vi "Color_Project.vi"() -> ()   [LabVIEW 2014]
uses:
  leitura de dados txt control.ctl
panel:
  out "L*a*b*":dbl[](array[numeric])
  out "r1":dbl[](array[numeric])
  out "Reflectance2":string[][](array[string])
  out "teste":i32[](array[numeric])
  out "IL Table":string[][](array[string])
  out "ILCols":i32
  out "ILRows":i32
  out "Selected illuminant":dbl[](array[numeric])
  out "Reflectance":i32[](array[numeric])
  out "Is CMF selected?":bool
  out "Is illuminant selected?":bool
  out "Intepoled iluminants":dbl[][](array[numeric])
  out "Selected\nCMF":dbl[][](array[numeric])
  out "cmf Index":dbl
  out "CMFCols":i32
  out "CMFRows":i32
  out "CMF Table":string[][](array[string])
  in  "Color Matching Function":string(combo)
  out "Illuminant Graph":T1(graph)
  out "LambdaInterval":dbl[](array[numeric])
  out "NeedInterpolation?":bool
  out "Selected illuminant index":dbl
  in  "Select Illuminant":T2
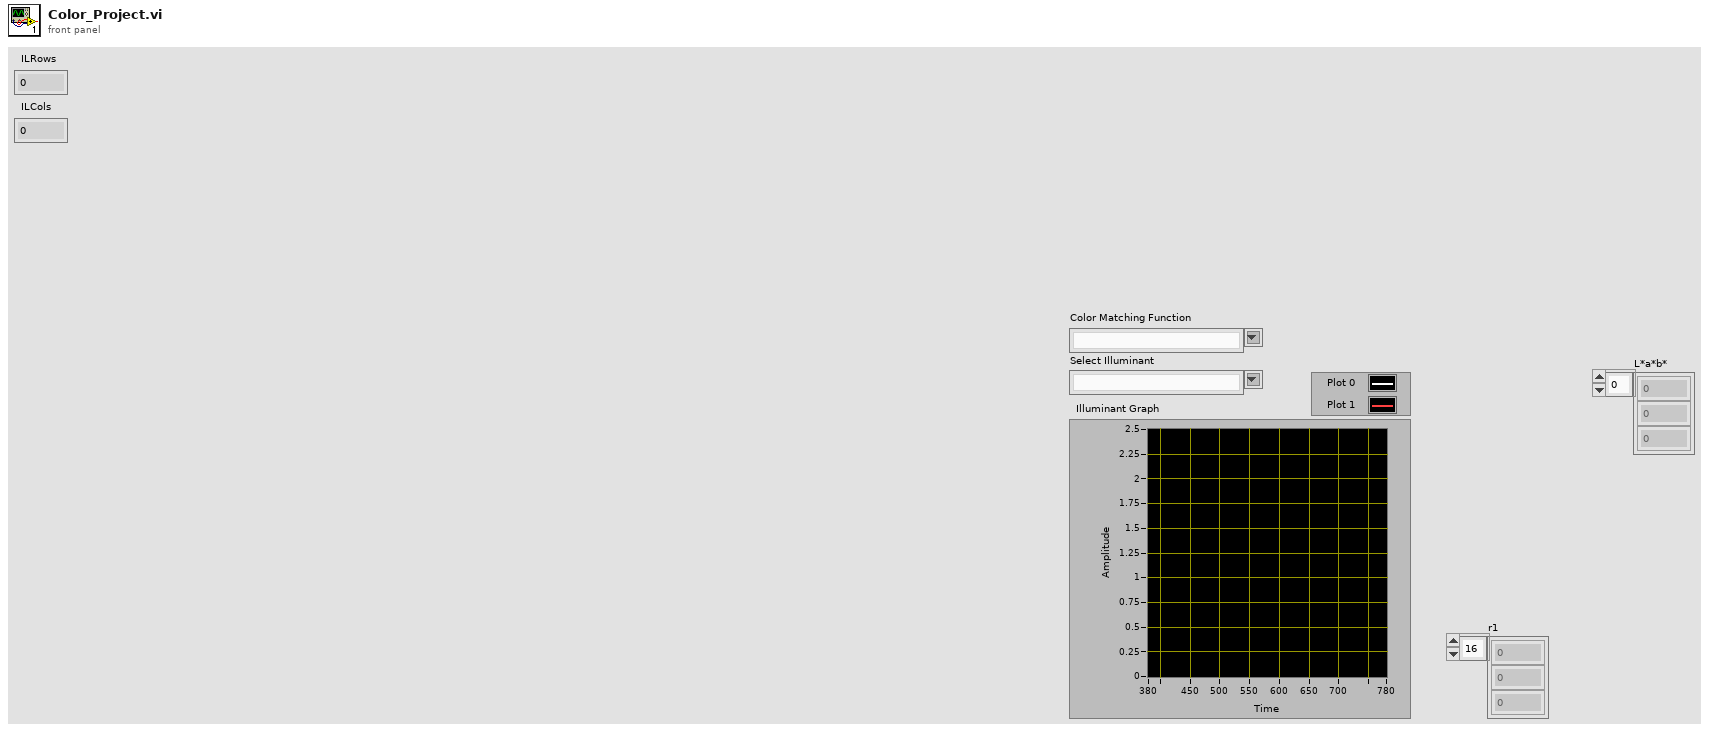
[diagram p1: front panel]
types:
  T1 = cluster{"GammaInterval":dbl[], "Interpolated":dbl[]}[]
  T2 = typedef "leitura de dados txt control.ctl" = string
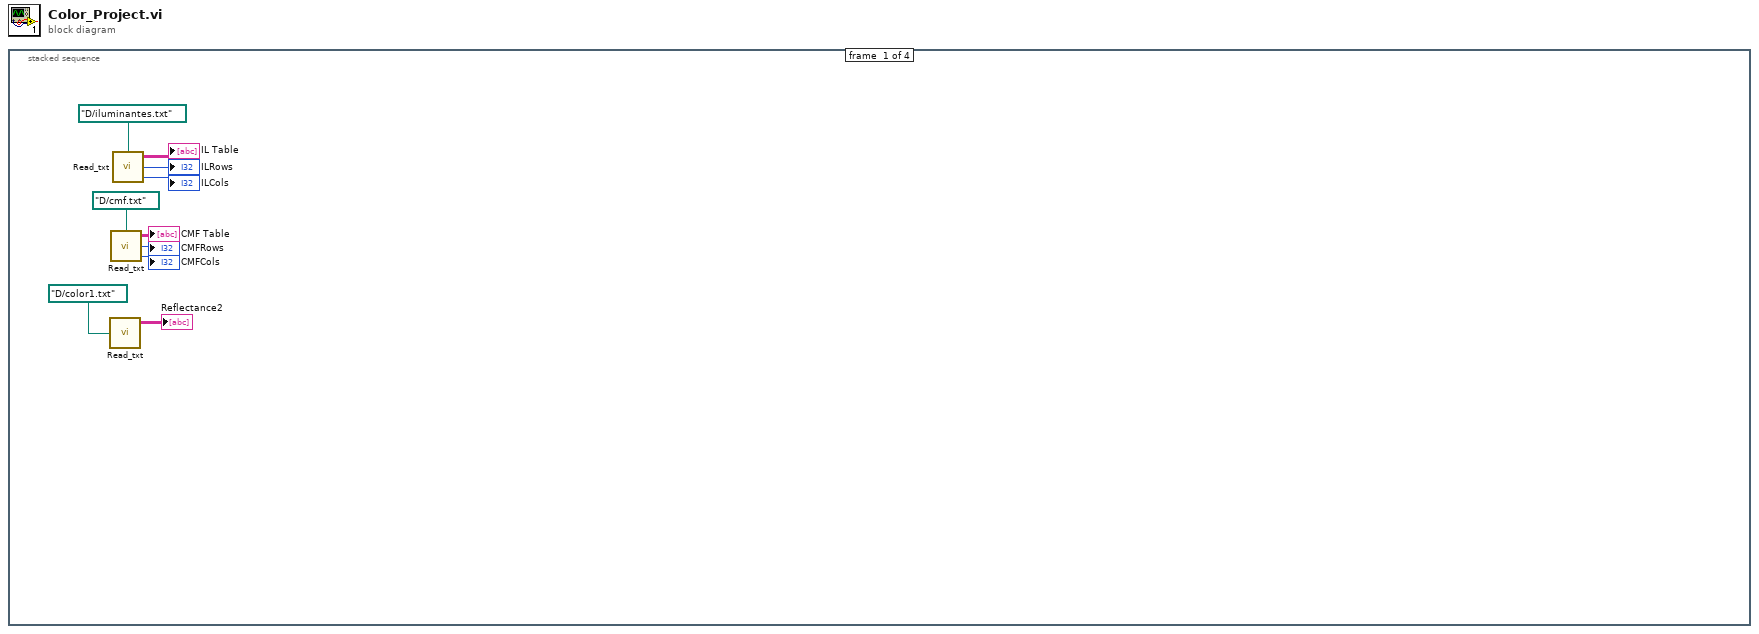
[diagram p0: block diagram]
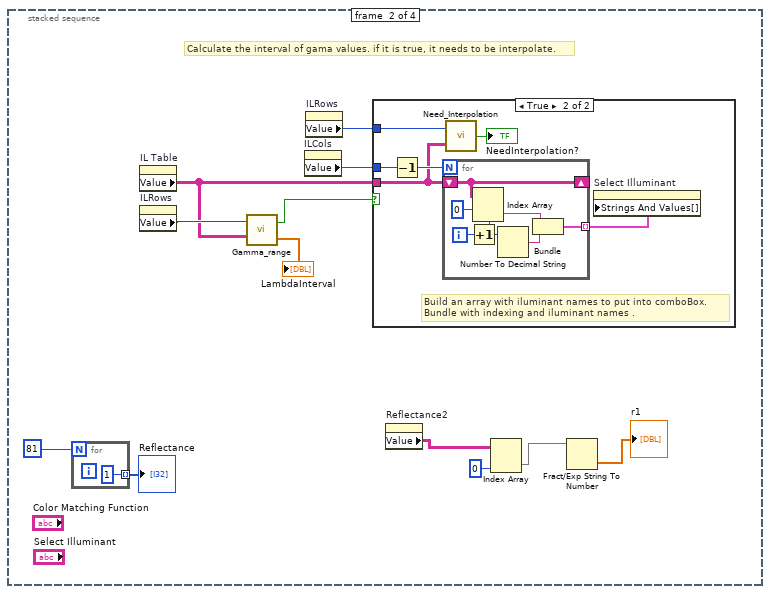
[diagram p2: hidden frame]
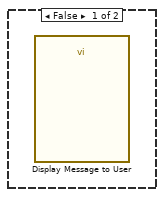
[diagram p3: hidden frame]
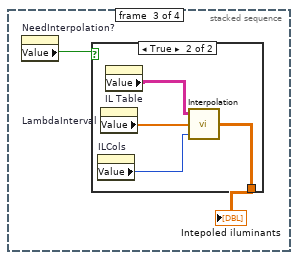
[diagram p4: hidden frame]
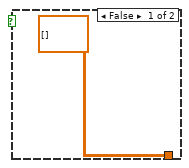
[diagram p5: hidden frame]
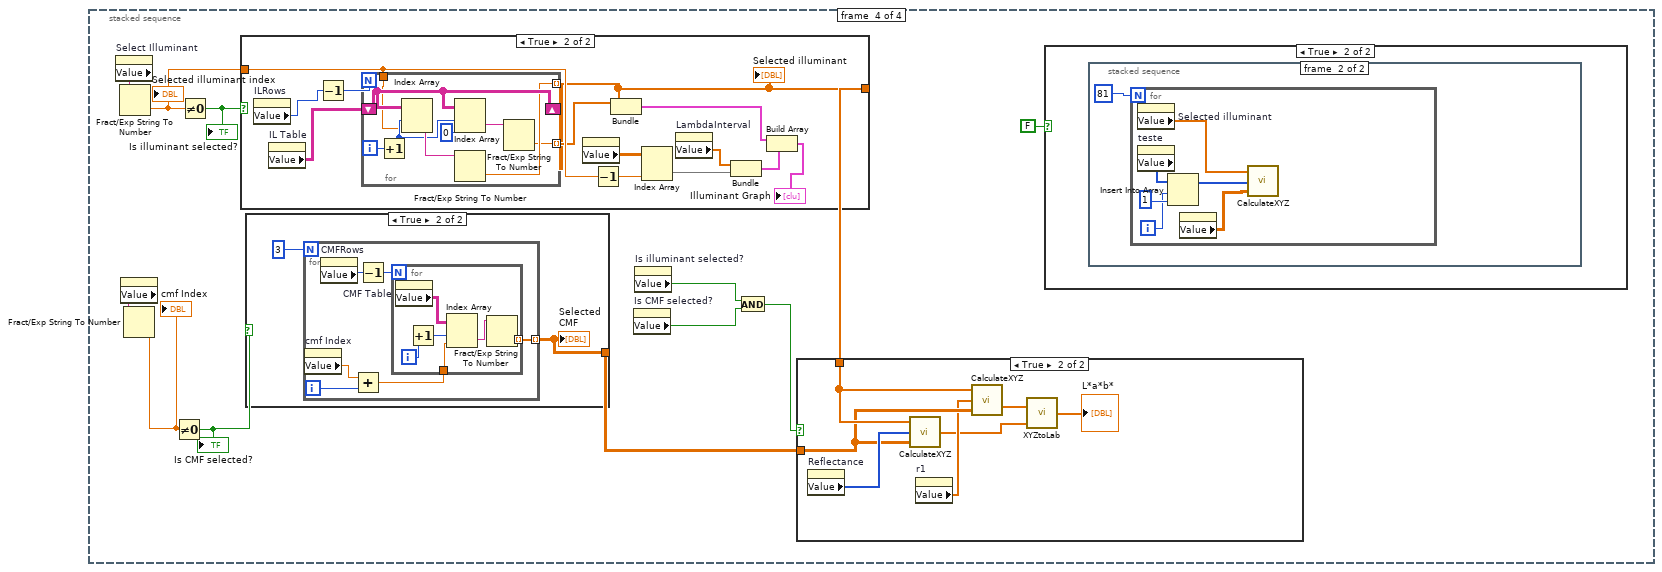
[diagram p6: hidden frame]
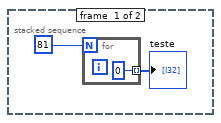
[diagram p8: hidden frame]
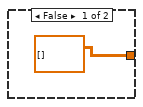
[diagram p10: hidden frame]
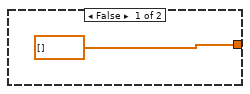
[diagram p11: hidden frame]
diagram:
  n1 = stacked-sequence {
    frame #0 {
      n2 = call "Read_txt.vi"("file path (dialog if empty)"=path "D:/color1.txt") -> ("Elements"=→"Reflectance2":string[][])  [unwired: 2 out]
      n3 = call "Read_txt.vi"("file path (dialog if empty)"=path "D:/cmf.txt") -> ("Elements"=→"CMF Table":string[][], "Rows"=→"CMFRows":i32, "Cols"=→"CMFCols":i32)
      n4 = call "Read_txt.vi"("file path (dialog if empty)"=path "D:/iluminantes.txt") -> ("Elements"=→"IL Table":string[][], "Rows"=→"ILRows":i32, "Cols"=→"ILCols":i32)
    }
    frame #1 {
      # "Calculate the interval of gama values. if it is true, it needs to be interpolate."
      n5 = for {
        N: 81 -> [_]
        tunnel: [1] -> w21 mode=indexing
      }
      "Reflectance" <- w21
      n6 = property on="IL Table" class="Arr (strict)"() -> ("Value"=w18:string[][])  [unwired: 2 in, 2 out]
      n7 = property on="ILRows" class="DigNum (strict)"() -> ("Value"=w19:i32)  [unwired: 2 in, 2 out]
      n8 = call "Gamma_range.vi"("Illuminant Table"=w18, "NumberOfRows"=w19) -> ("GammaInterval"=→"LambdaInterval":dbl[], "In range?"=w15:bool)
      n9 = property on="ILCols" class="DigNum (strict)"() -> ("Value"=w17:i32)  [unwired: 2 in, 2 out]
      n10 = property on="ILRows" class="DigNum (strict)"() -> ("Value"=w16:i32)  [unwired: 2 in, 2 out]
      n11 = case shown="True" w15 {
        tunnel: w18 -> [_ w24]
        tunnel: w17 -> [_ w25]
        tunnel: w16 -> [_ w23]
        frame False {
          n12 = call "Display Message to User"() -> ()  [unwired: 10 in, 2 out]
        }
        frame True {
          # "Build an array with iluminant names to put into comboBox.\nBundle with indexing and iluminant names ."
          n13 = Decrement(x=w25) -> (x-1=w27:i32)
          n14 = for {
            N: w27 -> [_]
            shift-right: [w33] -> _
            shift-left: w24 -> [w33]
            tunnel: [w29] -> w26 mode=indexing
            i -> [w35]
            n15 = Increment(x=w35) -> (x+1=w32:i32)
            n16 = Index Array(array=w33, index (row)=0, index (col)=w32) -> (element=w30:string)
            n17 = Number To Decimal String(number=w32) -> (decimal integer string=w31:string)  [unwired: 1 in]
            n18 = Bundle("String"=w30, w31) -> (w29:cluster{"String":string, string})  [unwired: 1 in]
          }
          n19 = call "Need_Interpolation.vi"("Matrix with txt"=w24, "Number of Rows"=w23) -> ("isNotFive?"=→"NeedInterpolation?":bool)
          n20 = property on="Select Illuminant" class="CmbBox (strict)"("Strings And Values[]"=w26) -> ()  [unwired: 2 in, 2 out]
        }
      }
      n21 = property on="Reflectance2" class="Arr (strict)"() -> ("Value"=w14:string[][])  [unwired: 2 in, 2 out]
      n22 = Index Array(array=w14, index (col)=0 ("disabled index (col)")) -> (element=w12:string[])  [unwired: 1 in]
      n23 = Fract/Exp String To Number(string=w12) -> (number=→"r1":dbl[])  [unwired: 3 in, 1 out]
    }
    frame #2 {
      n24 = property on="NeedInterpolation?" class="Bool (strict)"() -> ("Value"=w38:bool)  [unwired: 2 in, 2 out]
      n25 = case shown="True" w38 {
        tunnel: [dbl[][] [] w42] -> w37
        frame False {
        }
        frame True {
          n26 = property on="ILCols" class="DigNum (strict)"() -> ("Value"=w40:i32)  [unwired: 2 in, 2 out]
          n27 = property on="LambdaInterval" class="Arr (strict)"() -> ("Value"=w43:dbl[])  [unwired: 2 in, 2 out]
          n28 = property on="IL Table" class="Arr (strict)"() -> ("Value"=w41:string[][])  [unwired: 2 in, 2 out]
          n29 = call "Interpolation.vi"("Number of Columns"=w40, "Lambda Interval"=w43, "Illuminants"=w41) -> ("Interpolated"=w42:dbl[][])
        }
      }
      "Intepoled iluminants" <- w37
    }
    frame #3 {
      n30 = property on="Select Illuminant" class="CmbBox (strict)"() -> ("Value"=w51:T2)  [unwired: 2 in, 2 out]
      n31 = Fract/Exp String To Number(string=w51) -> (number=w50:dbl)  [unwired: 3 in, 1 out]
      "Selected illuminant index" <- w50
      n32 = property on="Color Matching Function" class="CmbBox"() -> ("Value"=w53:string)  [unwired: 2 in, 2 out]
      n33 = Fract/Exp String To Number(string=w53) -> (number=w54:dbl)  [unwired: 3 in, 1 out]
      "cmf Index" <- w54
      n34 = Not Equal To 0?(x=w54) -> (x != 0?=w52:bool)
      "Is CMF selected?" <- w52
      n35 = Not Equal To 0?(x=w50) -> (x != 0?=w55:bool)
      "Is illuminant selected?" <- w55
      n36 = case shown="True" w55 {
        tunnel: w50 -> [_ w97]
        tunnel: [dbl[] [] w91] -> w45
        frame False {
        }
        frame True {
          n37 = property on="ILRows" class="DigNum (strict)"() -> ("Value"=w90:i32)  [unwired: 2 in, 2 out]
          n38 = property on="IL Table" class="Arr (strict)"() -> ("Value"=w89:string[][])  [unwired: 2 in, 2 out]
          n39 = Decrement(x=w90) -> (x-1=w101:i32)
          n40 = for {
            N: w101 -> [_]
            shift-right: [w109] -> _
            shift-left: w89 -> [w109]
            tunnel: w97 -> [w102]
            tunnel: [w104] -> w91 mode=indexing
            tunnel: [w103] -> w93 mode=indexing
            i -> [w110]
            n41 = Increment(x=w110) -> (x+1=w105:i32)
            n42 = Index Array(array=w109, index (row)=w105, index (col)=w102) -> (element=w106:string)
            n43 = Index Array(array=w109, index (row)=w105, index (col)=0 ("disabled index (col)")) -> (element=w107:string)
            n44 = Fract/Exp String To Number(string=w106) -> (number=w104:dbl)  [unwired: 3 in, 1 out]
            n45 = Fract/Exp String To Number(string=w107) -> (number=w103:dbl)  [unwired: 3 in, 1 out]
          }
          "Selected illuminant" <- w91
          n46 = property on="Intepoled iluminants" class="Arr (strict)"() -> ("Value"=w95:dbl[][])  [unwired: 2 in, 2 out]
          n47 = Decrement(x=w97) -> (x-1=w96:dbl)
          n48 = Bundle(w93, w91) -> (w98:cluster{dbl[], dbl[]})  [unwired: 1 in]
          n49 = Index Array(array=w95, index (col)=w96) -> (element=w92:dbl[])  [unwired: 1 in]
          n50 = property on="LambdaInterval" class="Arr (strict)"() -> ("Value"=w94:dbl[])  [unwired: 2 in, 2 out]
          n51 = Bundle("Value"=w94, "Value"=w92) -> (w99:cluster{"Value":dbl[], "Value":dbl[]})  [unwired: 1 in]
          n52 = Build Array(w98, w99) -> (→"Illuminant Graph":cluster{"Value":dbl[], "Value":dbl[]}[])
        }
      }
      n53 = case shown="True" w52 {
        tunnel: [dbl[][] [] w74] -> w46
        frame False {
        }
        frame True {
          n54 = for {
            N: 3 -> [_]
            tunnel: [w78] -> w74 mode=indexing
            i -> [w80]
            n55 = property on="cmf Index" class="DigNum (strict)"() -> ("Value"=w81:dbl)  [unwired: 2 in, 2 out]
            n56 = property on="CMFRows" class="DigNum (strict)"() -> ("Value"=w77:i32)  [unwired: 2 in, 2 out]
            n57 = Add(x=w81, y=w80) -> (x+y=w79:dbl)
            n58 = Decrement(x=w77) -> (x-1=w76:i32)
            n59 = for {
              N: w76 -> [_]
              tunnel: w79 -> [w86]
              tunnel: [w82] -> w78 mode=indexing
              i -> [w85]
              n60 = property on="CMF Table" class="Arr (strict)"() -> ("Value"=w87:string[][])  [unwired: 2 in, 2 out]
              n61 = Increment(x=w85) -> (x+1=w84:i32)
              n62 = Index Array(array=w87, index (row)=w84, index (col)=w86) -> (element=w83:string)
              n63 = Fract/Exp String To Number(string=w83) -> (number=w82:dbl)  [unwired: 3 in, 1 out]
            }
          }
          "Selected\nCMF" <- w74
        }
      }
      n64 = property on="Is CMF selected?" class="Bool (strict)"() -> ("Value"=w48:bool)  [unwired: 2 in, 2 out]
      n65 = property on="Is illuminant selected?" class="Bool (strict)"() -> ("Value"=w49:bool)  [unwired: 2 in, 2 out]
      n66 = And(x=w49, y=w48) -> (x .and. y?=w47:bool)
      n67 = case shown="True" w47 {
        tunnel: w45 -> [_ w71]
        tunnel: w46 -> [_ w70]
        frame False {
        }
        frame True {
          n68 = property on="Reflectance" class="Arr (strict)"() -> ("Value"=w72:i32[])  [unwired: 2 in, 2 out]
          n69 = call "CalculateXYZ.vi"("CMF"=w70, "Reflectance"=w72, "Illuminant"=w71) -> ("XYZ"=w67:dbl[])
          n70 = property on="r1" class="Arr (strict)"() -> ("Value"=w69:dbl[])  [unwired: 2 in, 2 out]
          n71 = call "CalculateXYZ.vi"("CMF"=w70, "Reflectance"=w69, "Illuminant"=w71) -> ("XYZ"=w68:dbl[])
          n72 = call "XYZtoLab.vi"("XrYrZr"=w67, "XYZ"=w68) -> ("L*a*b*"=→"L*a*b*":dbl[])
        }
      }
      n73 = case shown="True" FALSE {
        frame False {
        }
        frame True {
          n74 = stacked-sequence {
            frame #0 {
              n75 = for {
                N: 81 -> [_]
                tunnel: [0] -> w56 mode=indexing
              }
              "teste" <- w56
            }
            frame #1 {
              n76 = for {
                N: 81 -> [_]
                i -> [w64]
                n77 = property on="Selected illuminant" class="Arr (strict)"() -> ("Value"=w62:dbl[])  [unwired: 2 in, 2 out]
                n78 = property on="teste" class="Arr (strict)"() -> ("Value"=w63:i32[])  [unwired: 2 in, 2 out]
                n79 = Insert Into Array(array=w63, index=w64, new element=1 ("new element/subarray")) -> (w61:i32[])
                n80 = property on="Selected\nCMF" class="Arr (strict)"() -> ("Value"=w60:dbl[][])  [unwired: 2 in, 2 out]
                n81 = call "CalculateXYZ.vi"("CMF"=w60, "Reflectance"=w61, "Illuminant"=w62) -> ()  [unwired: 1 out]
              }
            }
          }
        }
      }
    }
  }
